vi "Unitary_Test_Get.vi"() -> (0 "Test_passed":bool)   [LabVIEW 2014]
panel:
  in  "Expected values":string[](array[string])=["0", "\"hola\"", "0.000000", "false", "0.000000"]
  out "error 2 must FAIL":errorcluster
  in  "bad variables":string[](array[string])=["fakevar", "stringout", "time"]
  out "values":string[](array[string])=["0", "\"hola\"", "0.000000", "false", "0.000000"]
  in  "variables":string[](array[string])=["intout", "stringout", "time", "booleanout", "doubleout"]
  out "error 1 must be OK":errorcluster
  out "hidden3":errorcluster
  out "hidden":errorcluster
  in  "Experience ID1":string="TestOK"
  out "Test_OK":bool[](array[boolean])=[FALSE, TRUE]
  # "Test basic methods with some testing plant"
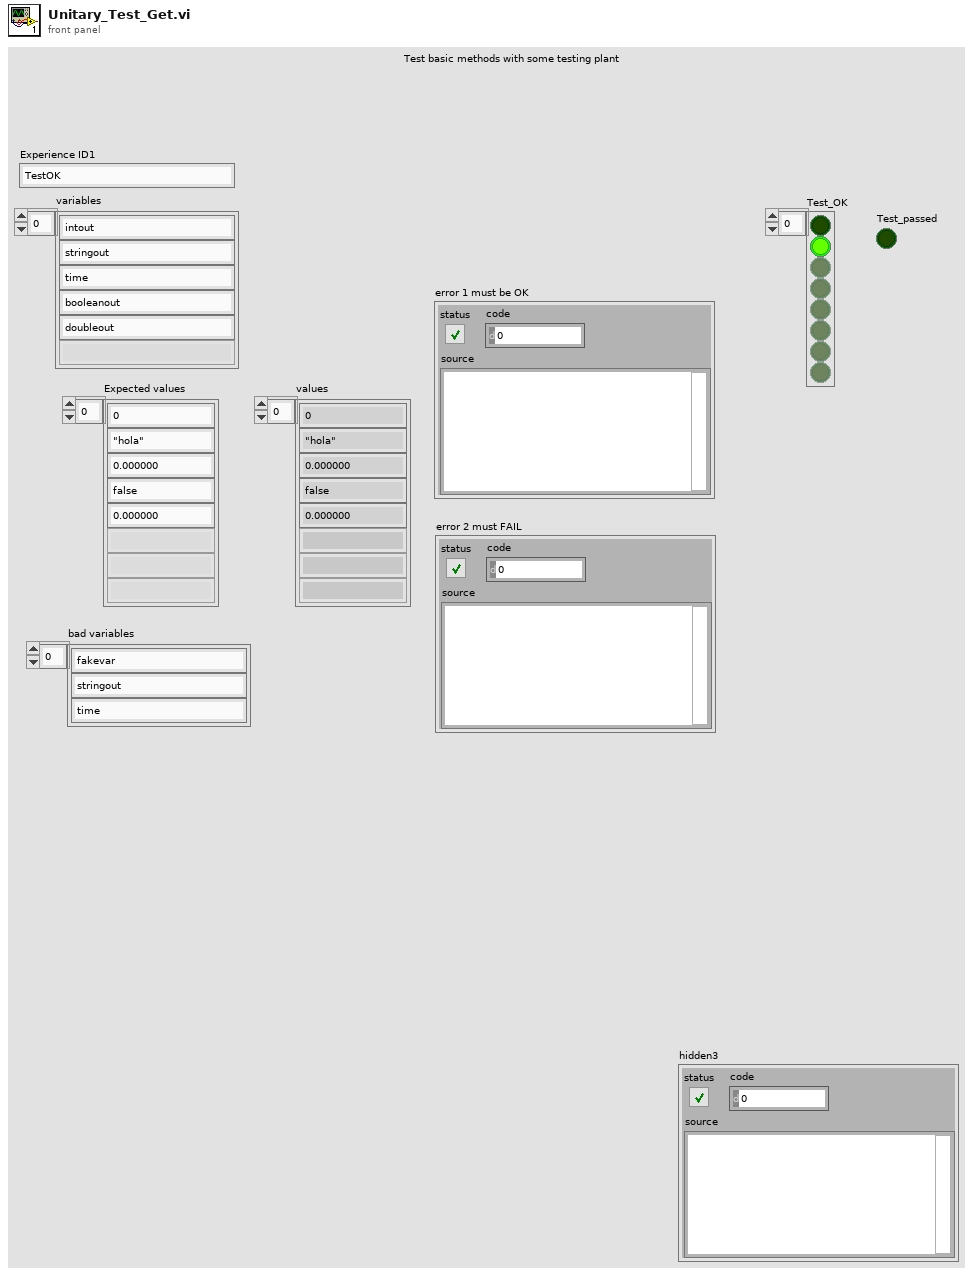
[diagram p1: front panel]
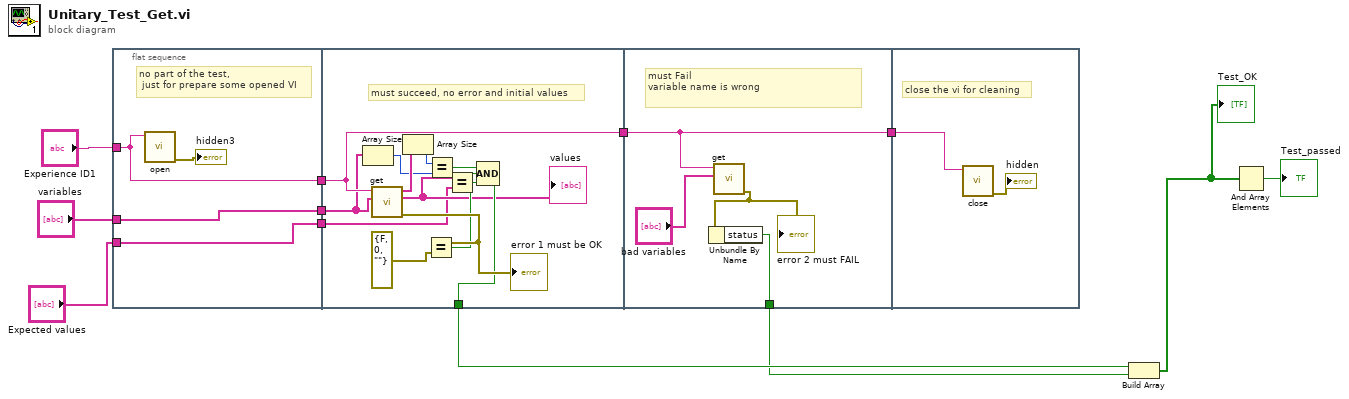
[diagram p0: block diagram]
diagram:
  n1 = flat-sequence {
    tunnel: "Experience ID1" -> [w15]
    tunnel: [w15] -> w8
    tunnel: [w14] -> w7
    tunnel: "variables" -> [w14]
    tunnel: [w13] -> w2
    tunnel: "Expected values" -> [w13]
    tunnel: [w21] -> w5
    tunnel: [w25] -> w10
    tunnel: w8 -> [w21]
    tunnel: w7 -> [w20]
    tunnel: w2 -> [w23]
    tunnel: w5 -> [w33]
    tunnel: [w33] -> w4
    tunnel: [w31] -> w3
    tunnel: w4 -> [w34]
    frame #0 {
      # "no part of the test,\n just for prepare some opened VI"
      n2 = call "open.vi"("Experience ID"=w15) -> ("error out"=→"hidden3":errorcluster)  [unwired: 8 in, 2 out]
    }
    frame #1 {
      # "must succeed, no error and initial values"
      n3 = Array Size(array=w20) -> (size(s)=w18:i32)
      n4 = call "get.vi"("variables"=w20, "Experience ID"=w21) -> ("error out"=w28:errorcluster, "values"=w24:string[], "names"=w19:string[])  [unwired: 7 in]
      "error 1 must be OK" <- w28
      "values" <- w24
      n5 = Array Size(array=w19) -> (size(s)=w17:i32)
      n6 = Equal?(x=w28, y=errorcluster {"status"=FALSE, "code"=0, "source"=""} ("error out")) -> (x = y?=w26:bool)
      n7 = Equal?(x=w17, y=w18) -> (x = y?=w27:bool)
      n8 = Equal?(x=w24, y=w23) -> (x = y?=w22:bool)
      n9 = Compound Arithmetic op=AND(w27, w26, w22) -> (w25:bool)
    }
    frame #2 {
      # "must Fail\nvariable name is wrong"
      n10 = call "get.vi"("variables"="bad variables", "Experience ID"=w33) -> ("error out"=w30:errorcluster)  [unwired: 7 in, 2 out]
      "error 2 must FAIL" <- w30
      n11 = Unbundle By Name(w30) -> ("status"=w31:bool)
    }
    frame #3 {
      # "close the vi for cleaning"
      n12 = call "close.vi"("Experience ID"=w34) -> ("error out"=→"hidden":errorcluster)  [unwired: 10 in]
    }
  }
  n13 = Build Array(w10, w3) -> (w9:bool[])
  "Test_OK" <- w9
  n14 = And Array Elements(Boolean array=w9) -> (logical AND=→"Test_passed":bool)
